vi "Hydra.vi"() -> ()   [LabVIEW 2019]
uses:
  Global Variables/Global_Variables.vi
panel:
  in  "Press Transducer Cal":u16(ring) items=["Low Pressure", "High Pressure"]
  in  "Cal Add":bool
  out "Error Code":i32
  out "Error Description":string
  out "Data":string[][](table)
  in  "Check":bool
  in  "Start Test":bool
  in  "Stop Test":bool
  in  "Quit":bool
  out "Channel_Config":string[][](table)
  in  "Add Button":bool
  in  "Cal":bool
  in  "Range":u16(ring)
  in  "Type":u16(ring)
  in  "Name":string
  in  "Channel":u16(ring)
  out "Status":string
  in  "Test Name":string
  in  "COM Port - Hydra":refnum<visa-resource-name>
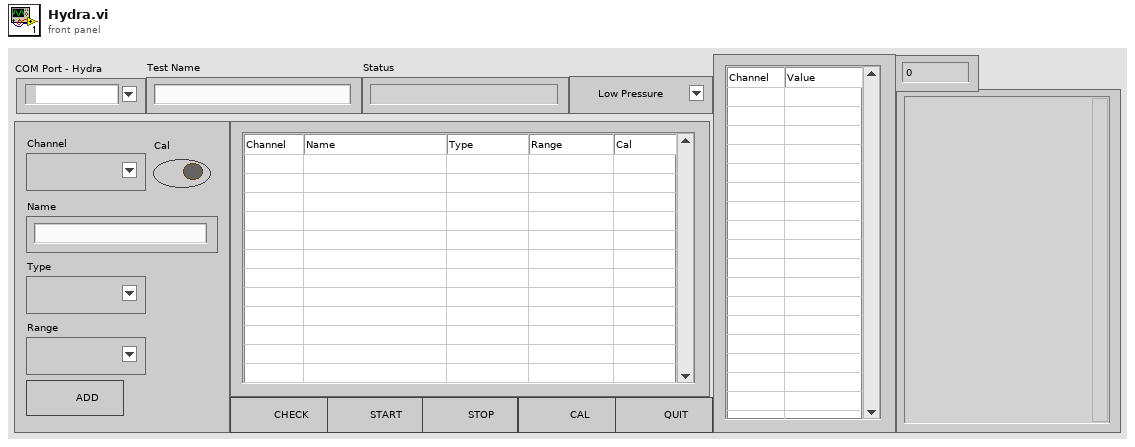
[diagram p1: front panel]
types:
  T1 = enum16{"Initialize", "Wait for Config", "Calibration", "Test", "Close"}
  T2 = enum8{"Enabled", "Disabled", "Disabled and Grayed Out"}
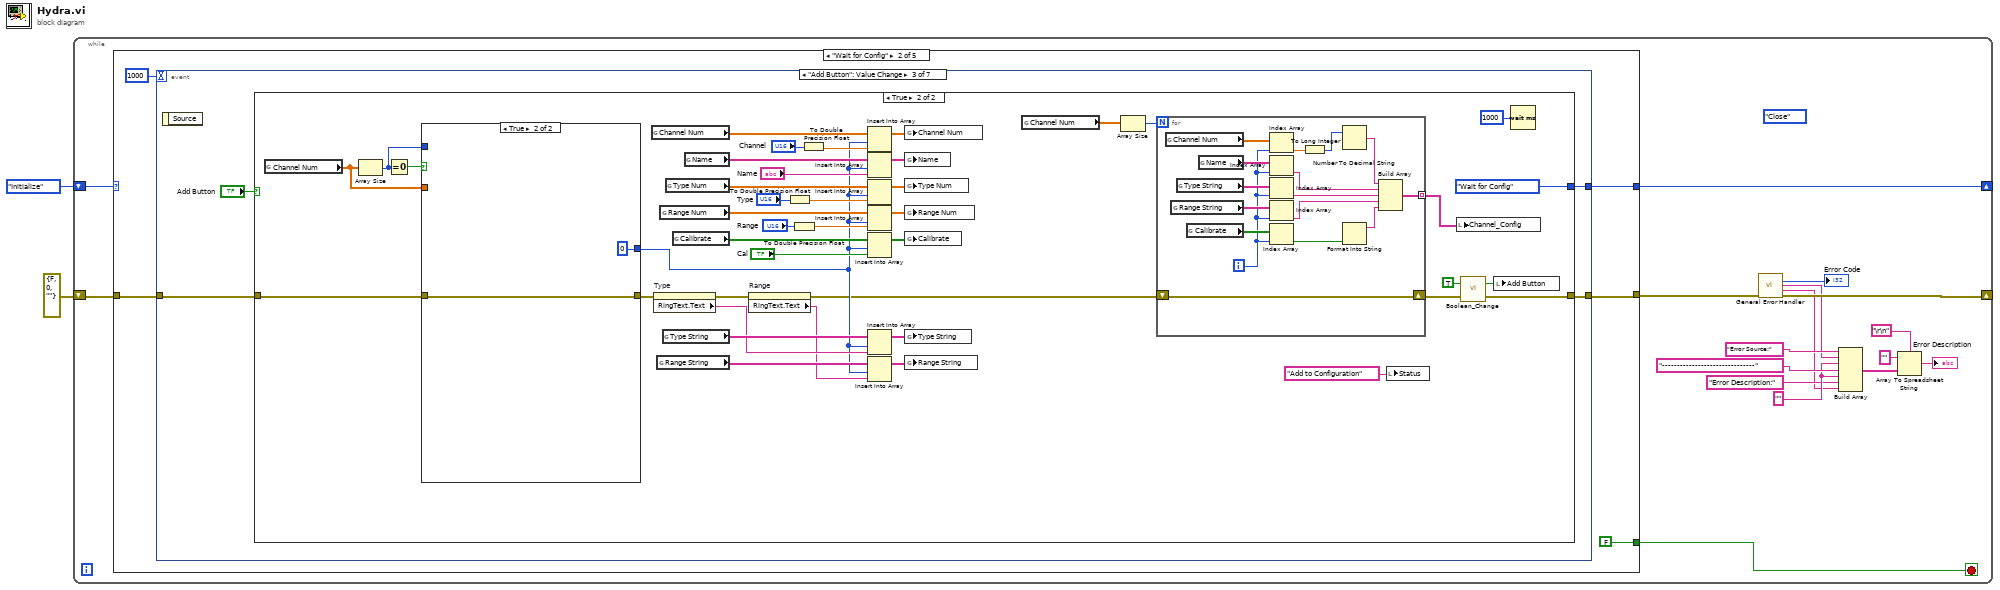
[diagram p0: block diagram]
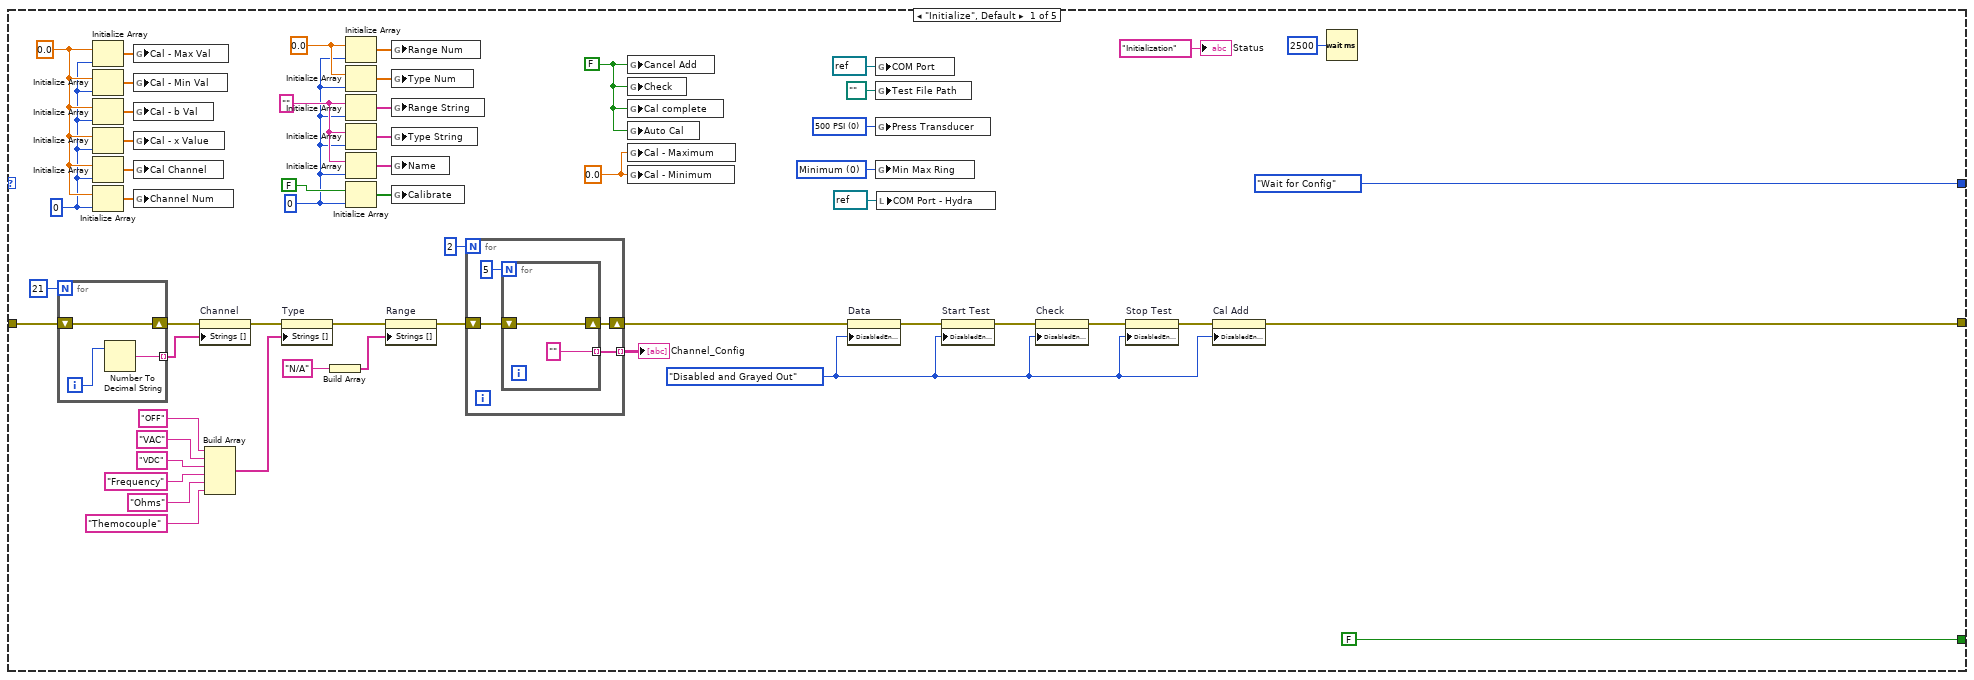
[diagram p2: hidden frame]
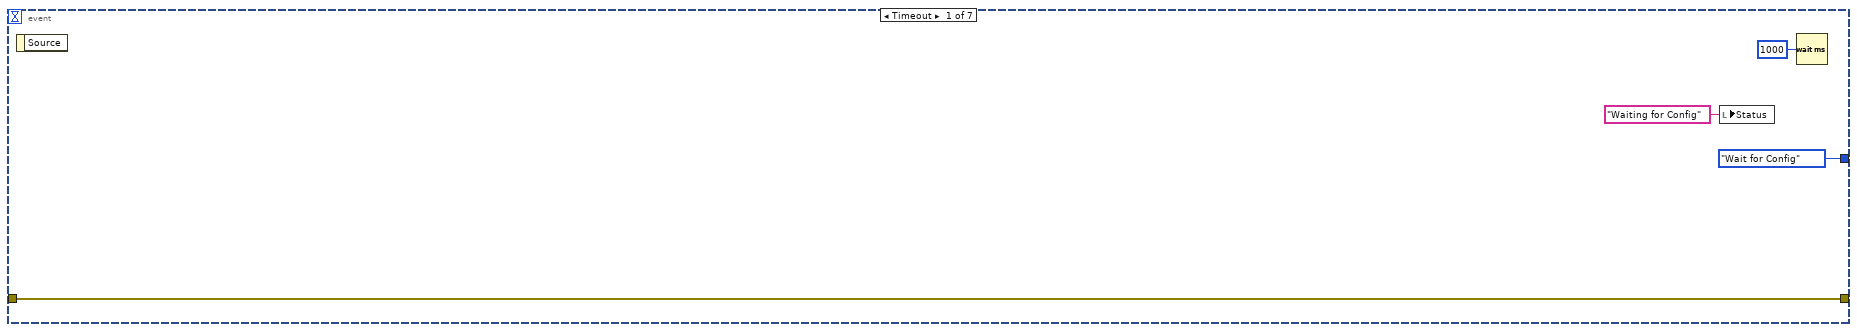
[diagram p3: hidden frame]
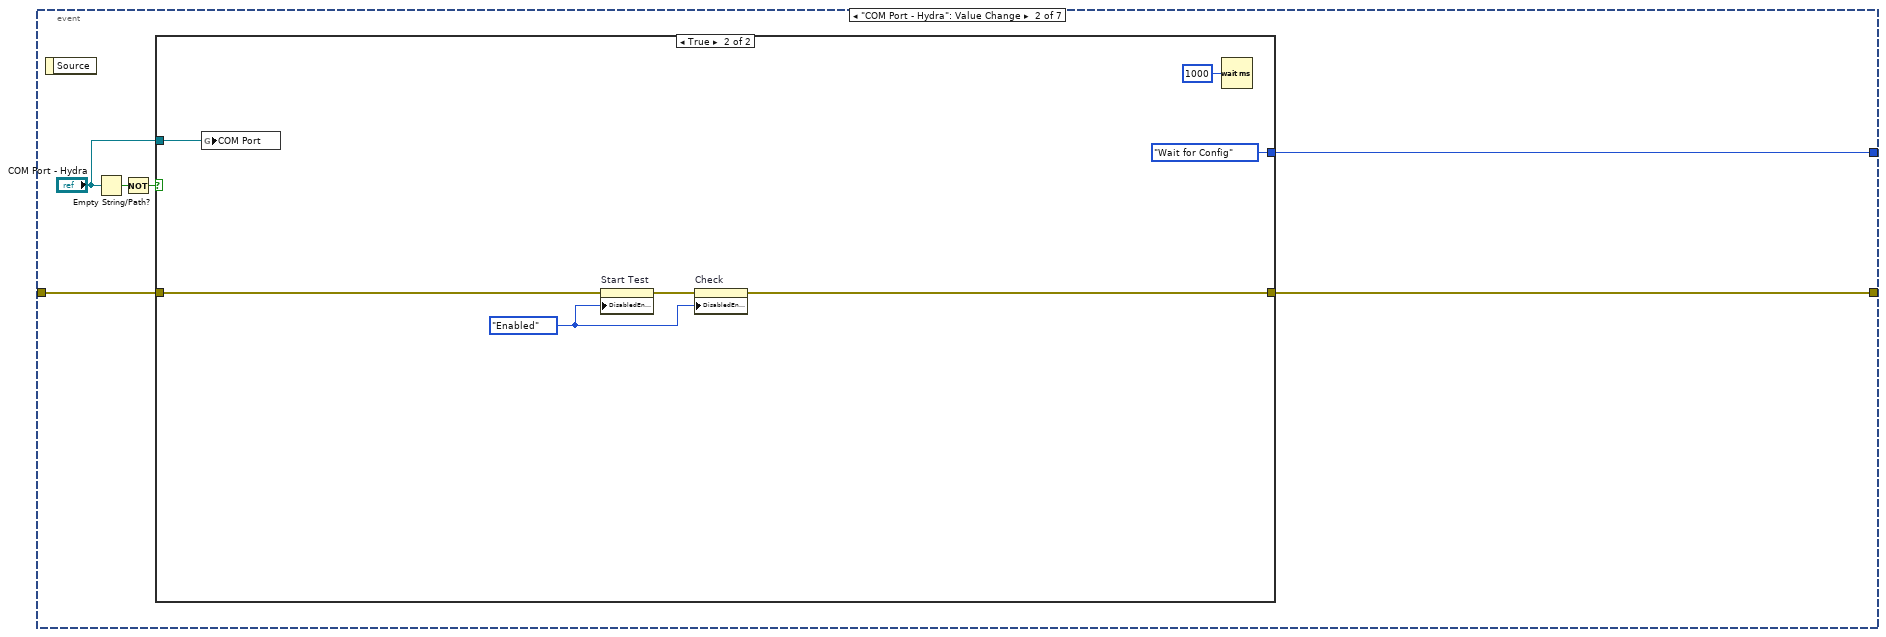
[diagram p4: hidden frame]
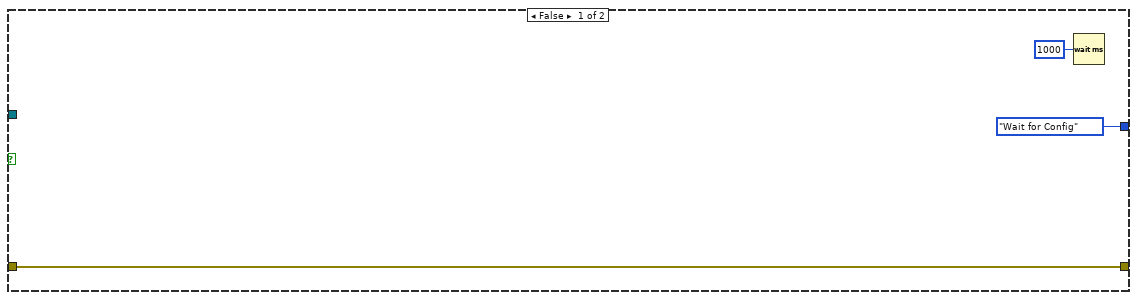
[diagram p5: hidden frame]
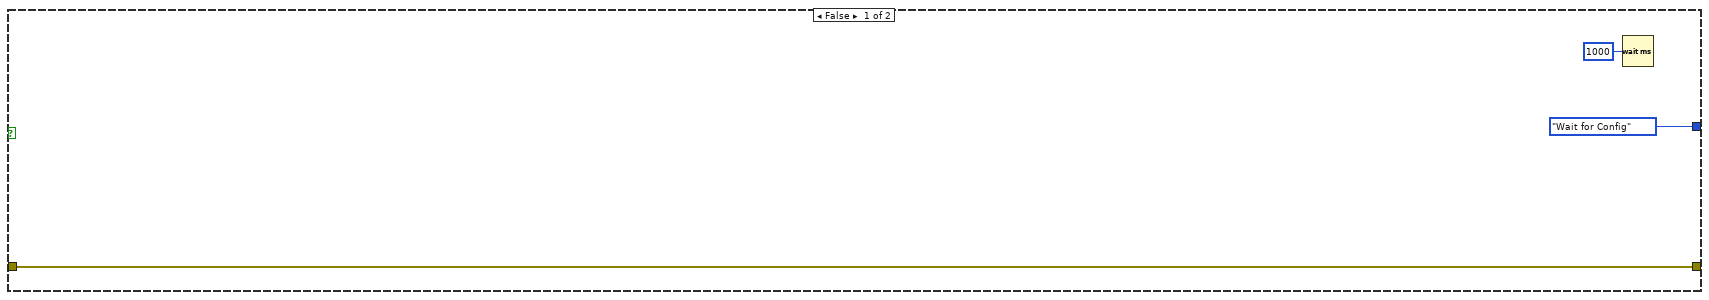
[diagram p6: hidden frame]
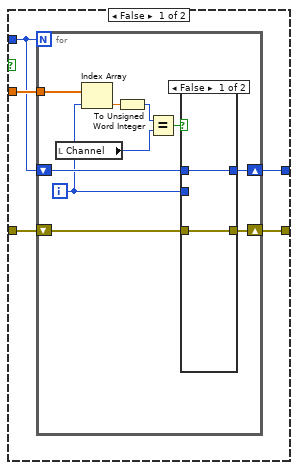
[diagram p7: hidden frame]
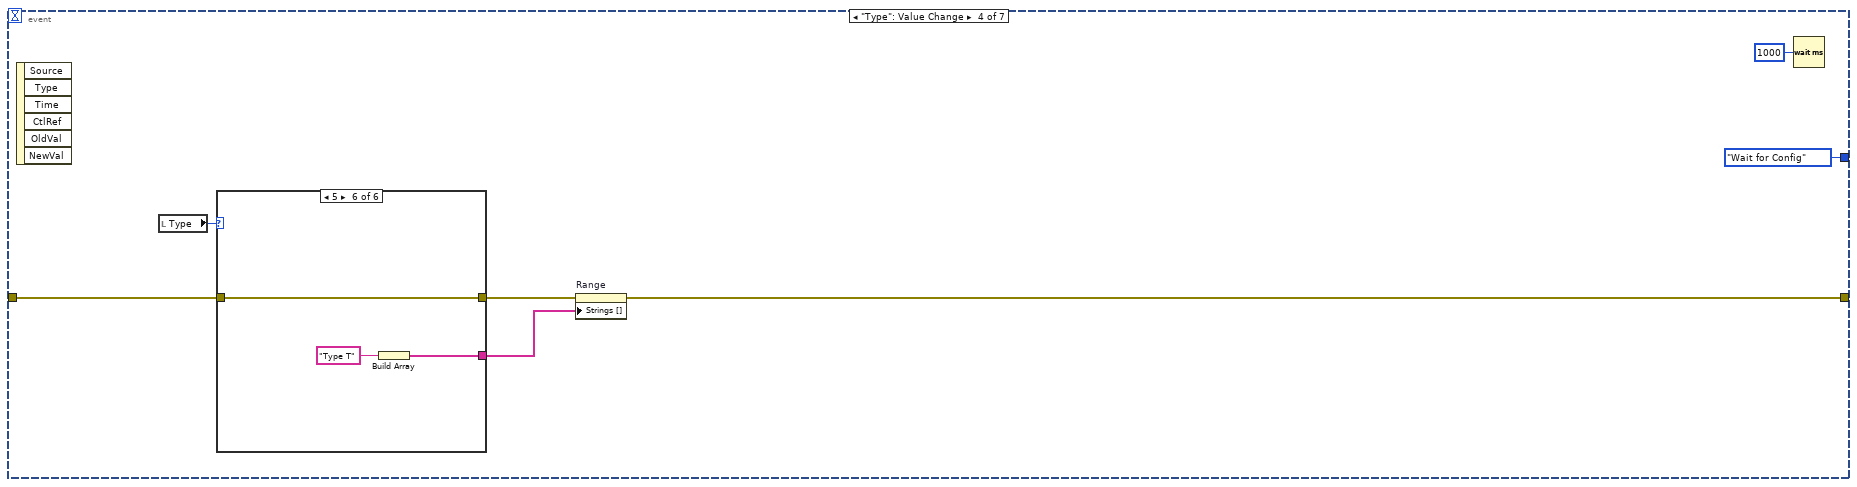
[diagram p9: hidden frame]
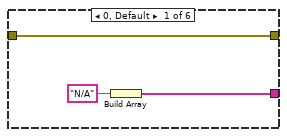
[diagram p10: hidden frame]
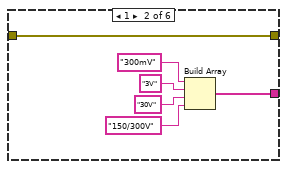
[diagram p11: hidden frame]
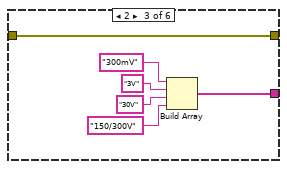
[diagram p12: hidden frame]
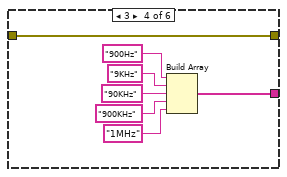
[diagram p13: hidden frame]
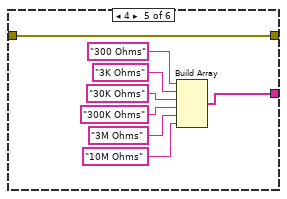
[diagram p14: hidden frame]
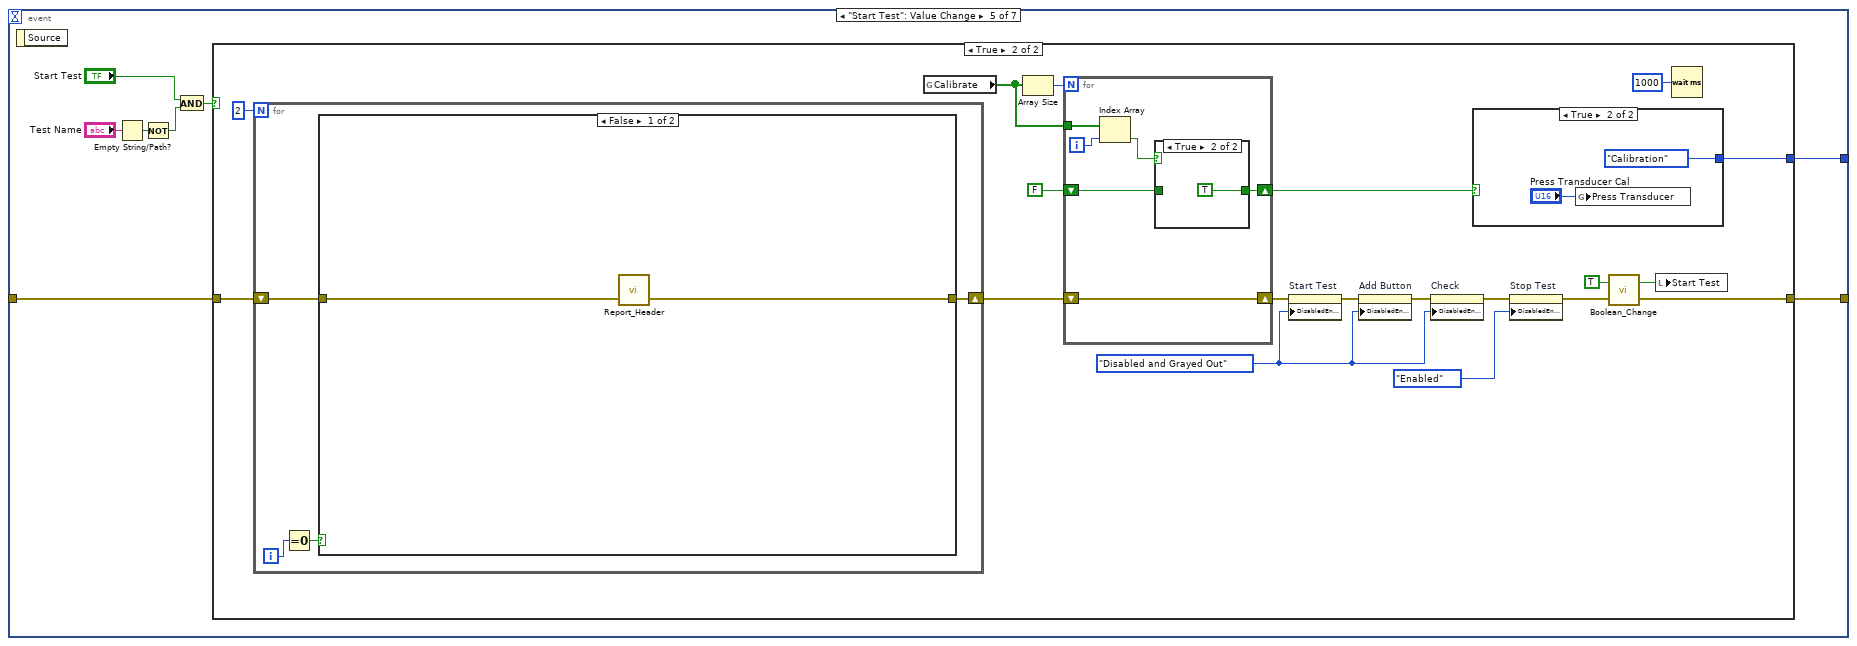
[diagram p15: hidden frame]
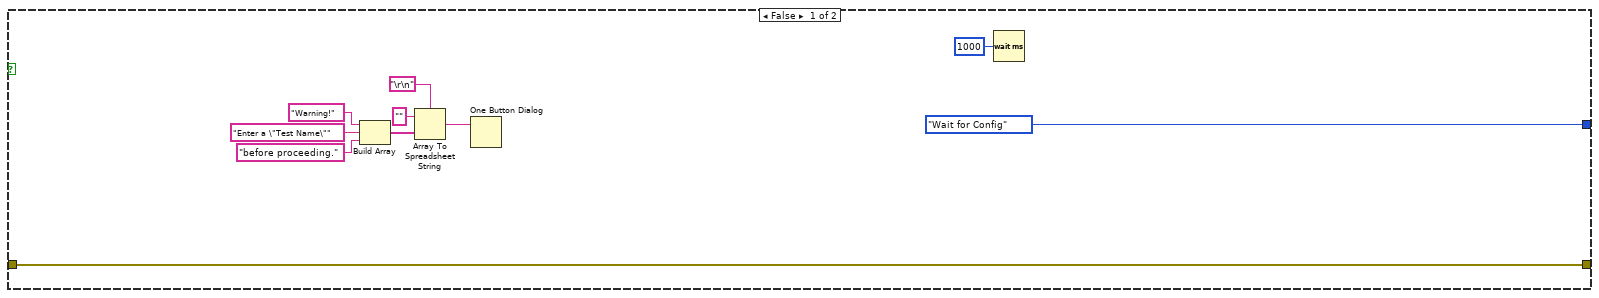
[diagram p16: hidden frame]
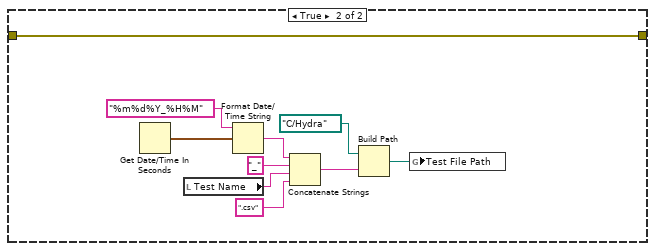
[diagram p17: hidden frame]
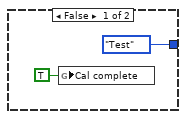
[diagram p18: hidden frame]
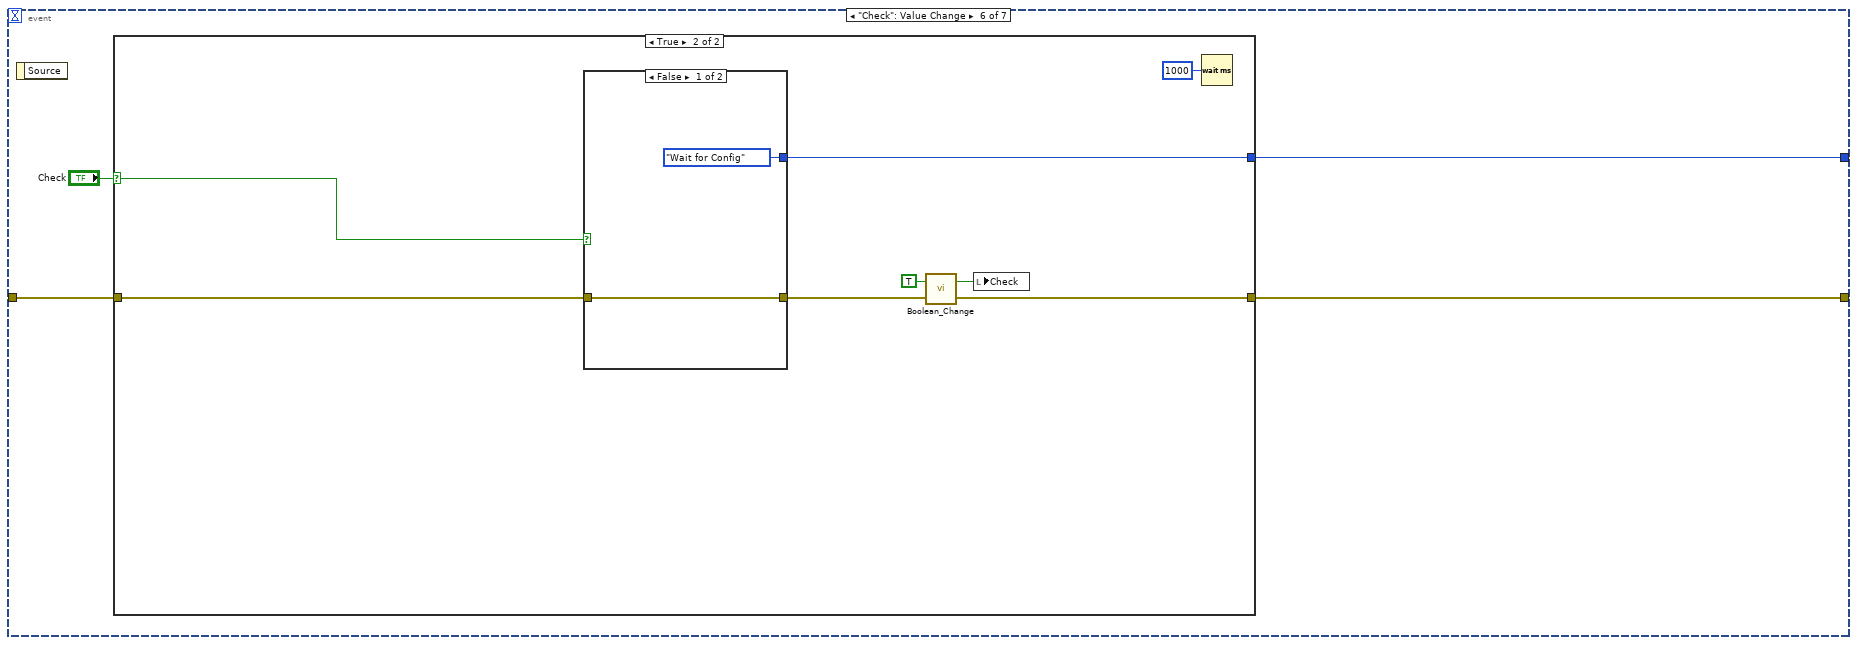
[diagram p20: hidden frame]
diagram:
  n1 = while {
    shift-right: [w15] -> _
    shift-left: errorcluster {"status"=FALSE, "code"=0, "source"=""} ("error constant") -> [w18]
    shift-right: [w3] -> _
    shift-left: T1."Initialize" -> [w19]
    stop <- w17 stop-if-true
    (unwired) T1."Close"
    w10 = ""
    n2 = case shown="\"Wait for Config\"" w19 {
      tunnel: w18 -> [w70 w86 w333 w594 w629]
      tunnel: [w45 w83 w331 w593 w629] -> w16
      tunnel: [FALSE FALSE FALSE FALSE TRUE] -> w17
      tunnel: [T1."Wait for Config" w84 w330 w592 T1."Close"] -> w3
      frame "Initialize", Default {
        w21 = u16 0 items=["Minimum", "Maximum"] ("Min Max Ring")
        w22 = u16 0 items=["500 PSI", "1000 PSI"] ("Press Transducer")
        w25 = FALSE ("Cancel Add")
        w26 = 0.0 ("Cal - Minimum")
        w34 = ""
        w36 = 0.0 ("element")
        w33 = 0 ("dimension size")
        w43 = 0 ("dimension size")
        w44 = 0.0 ("element")
        w46 = T2."Disabled and Grayed Out" ("Disabled")
        n3 = for {
          N: 21 -> [_]
          shift-right: [w82] -> w69
          shift-left: w70 -> [w82]
          tunnel: [w80] -> w68 mode=indexing
          i -> [w81]
          n4 = Number To Decimal String(number=w81) -> (decimal integer string=w80:string)  [unwired: 1 in]
        }
        n5 = Initialize Array(w44, w43) -> (w42:dbl[])
        n6 = Initialize Array(w44, w43) -> (w41:dbl[])
        n7 = Initialize Array(w44, w43) -> (w40:dbl[])
        n8 = Initialize Array(w44, w43) -> (w39:dbl[])
        n9 = Initialize Array(w44, w43) -> (w38:dbl[])
        n10 = Initialize Array(w44, w43) -> (w37:dbl[])
        n11 = global write "Global_Variables.vi" "Cal - Max Val"(w42) -> ()
        n12 = global write "Global_Variables.vi" "Cal - Min Val"(w41) -> ()
        n13 = global write "Global_Variables.vi" "Cal - b Val"(w40) -> ()
        n14 = global write "Global_Variables.vi" "Cal - x Value"(w39) -> ()
        n15 = global write "Global_Variables.vi" "Cal Channel"(w38) -> ()
        n16 = global write "Global_Variables.vi" "Channel Num"(w37) -> ()
        n17 = property on="Channel" class="Ring (strict)"(error in=w69, "Strings []"=w68) -> (error out=w61:errorcluster)  [unwired: 1 in, 1 out]
        n18 = Build Array("OFF", "VAC", "VDC", "Frequency", "Ohms", "Themocouple") -> (w60:string[])
        n19 = property on="Type" class="Ring (strict)"(error in=w61, "Strings []"=w60) -> (error out=w59:errorcluster)  [unwired: 1 in, 1 out]
        n20 = Build Array("N/A") -> (w57:string[])
        n21 = Initialize Array(w36, w33) -> (w32:dbl[])
        n22 = Initialize Array(w36, w33) -> (w31:dbl[])
        n23 = Initialize Array(w34, w33) -> (w30:string[])
        n24 = Initialize Array(w34, w33) -> (w29:string[])
        n25 = Initialize Array(w34, w33) -> (w28:string[])
        n26 = Initialize Array(FALSE, w33) -> (w27:bool[])
        n27 = property on="Range" class="Ring (strict)"(error in=w59, "Strings []"=w57) -> (error out=w56:errorcluster)  [unwired: 1 in, 1 out]
        n28 = global write "Global_Variables.vi" "Range Num"(w32) -> ()
        n29 = global write "Global_Variables.vi" "Type Num"(w31) -> ()
        n30 = global write "Global_Variables.vi" "Range String"(w30) -> ()
        n31 = global write "Global_Variables.vi" "Type String"(w29) -> ()
        n32 = global write "Global_Variables.vi" "Name"(w28) -> ()
        n33 = global write "Global_Variables.vi" "Calibrate"(w27) -> ()
        n34 = for {
          N: 2 -> [_]
          shift-right: [w75] -> w53
          shift-left: w56 -> [w76]
          tunnel: [w74] -> w54 mode=indexing
          n35 = for {
            N: 5 -> [_]
            shift-right: [w79] -> w75
            shift-left: w76 -> [w79]
            tunnel: [""] -> w74 mode=indexing
          }
        }
        "Channel_Config" <- w54
        n36 = global write "Global_Variables.vi" "Cancel Add"(w25) -> ()
        n37 = global write "Global_Variables.vi" "Check"(w25) -> ()
        n38 = global write "Global_Variables.vi" "Cal complete"(w25) -> ()
        n39 = global write "Global_Variables.vi" "Auto Cal"(w25) -> ()
        n40 = global write "Global_Variables.vi" "Cal - Maximum"(w26) -> ()
        n41 = global write "Global_Variables.vi" "Cal - Minimum"(w26) -> ()
        n42 = property on="Data" class="Tbl (strict)"(error in=w53, "DisabledEnum"=w46) -> (error out=w52:errorcluster)  [unwired: 1 in, 1 out]
        n43 = global write "Global_Variables.vi" "COM Port"(refnum<visa-resource-name> refnum ("COM Port")) -> ()
        n44 = global write "Global_Variables.vi" "Test File Path"(path "" ("Test File Path")) -> ()
        n45 = global write "Global_Variables.vi" "Press Transducer"(w22) -> ()
        n46 = global write "Global_Variables.vi" "Min Max Ring"(w21) -> ()
        n47 = local write "COM Port - Hydra"(refnum<visa-resource-name> refnum ("COM Port - Hydra")) -> ()
        n48 = property on="Start Test" class="Bool (strict)"(error in=w52, "DisabledEnum"=w46) -> (error out=w51:errorcluster)  [unwired: 1 in, 1 out]
        n49 = property on="Check" class="Bool (strict)"(error in=w51, "DisabledEnum"=w46) -> (error out=w50:errorcluster)  [unwired: 1 in, 1 out]
        n50 = property on="Stop Test" class="Bool (strict)"(error in=w50, "DisabledEnum"=w46) -> (error out=w47:errorcluster)  [unwired: 1 in, 1 out]
        n51 = property on="Cal Add" class="Bool (strict)"(error in=w47, "DisabledEnum"=w46) -> (error out=w45:errorcluster)  [unwired: 1 in, 1 out]
        n52 = Wait (ms)(milliseconds to wait=u32 2500) -> ()  [unwired: 1 out]
        "Status" <- "Initialization" ("Status")
      }
      frame "Wait for Config" {
        n53 = event shown="[2] \"Add Button\": Value Change" {
          selector: _ -> [_ _ _ _ _ _ _]
          dyn-events: _ -> [_ _ _ _ _ _ _]
          timeout: 1000 -> [_ _ _ _ _ _ _]
          tunnel: w86 -> [w91 w96 w110 w199 w237 w300 w321]
          tunnel: [T1."Wait for Config" w97 w108 T1."Wait for Config" w236 w301 w320] -> w84
          tunnel: [w91 w95 w109 w195 w234 w299 w319] -> w83
          event Timeout {
            n54 = event-data() -> ()  [unwired: 1 in, 1 out]
            n55 = local write "Status"("Waiting for Config" ("Status")) -> ()
            n56 = Wait (ms)(milliseconds to wait=u32 1000) -> ()  [unwired: 1 out]
          }
          event "COM Port - Hydra": Value Change {
            n57 = event-data() -> ()  [unwired: 1 in, 1 out]
            n58 = Empty String/Path?(string/path="COM Port - Hydra") -> (empty?=w93:bool)
            n59 = Not(x=w93) -> (.not. x?=w92:bool)
            n60 = case shown="True" w92 {
              tunnel: [T1."Wait for Config" T1."Wait for Config"] -> w97
              tunnel: w96 -> [w99 w107]
              tunnel: [w99 w105] -> w95
              tunnel: "COM Port - Hydra" -> [_ w101]
              frame False {
                n61 = Wait (ms)(milliseconds to wait=u32 1000) -> ()  [unwired: 1 out]
              }
              frame True {
                w103 = T2."Enabled" ("Disabled")
                n62 = global write "Global_Variables.vi" "COM Port"(w101) -> ()
                n63 = property on="Start Test" class="Bool (strict)"(error in=w107, "DisabledEnum"=w103) -> (error out=w106:errorcluster)  [unwired: 1 in, 1 out]
                n64 = property on="Check" class="Bool (strict)"(error in=w106, "DisabledEnum"=w103) -> (error out=w105:errorcluster)  [unwired: 1 in, 1 out]
                n65 = Wait (ms)(milliseconds to wait=u32 1000) -> ()  [unwired: 1 out]
              }
            }
          }
          event "Add Button": Value Change {
            n66 = event-data() -> ()  [unwired: 1 in, 1 out]
            n67 = case shown="True" "Add Button" {
              tunnel: w110 -> [w114 w154]
              tunnel: [w114 w117] -> w109
              tunnel: [T1."Wait for Config" T1."Wait for Config"] -> w108
              frame False {
                n68 = Wait (ms)(milliseconds to wait=u32 1000) -> ()  [unwired: 1 out]
              }
              frame True {
                n69 = global read "Global_Variables.vi" "Channel Num"() -> (w155:dbl[])
                n70 = Array Size(array=w155) -> (size(s)=w153:i32)
                n71 = Equal To 0?(x=w153) -> (x = 0?=w156:bool)
                n72 = case shown="True" w156 {
                  tunnel: w155 -> [w177 _]
                  tunnel: w154 -> [w176 w193]
                  tunnel: [w175 w193] -> w144
                  tunnel: w153 -> [w173 _]
                  tunnel: [w174 0] -> w131
                  frame False {
                    n73 = for {
                      N: w173 -> [_]
                      tunnel: w177 -> [w187]
                      shift-right: [w181] -> w175
                      shift-left: w176 -> [w182]
                      shift-right: [w179] -> w174
                      shift-left: w173 -> [w180]
                      i -> [w178]
                      n74 = local read "Channel"() -> (w184:u16)
                      n75 = Index Array(array=w187, index=w178) -> (element=w186:dbl)
                      n76 = To Unsigned Word Integer(number=w186) -> (unsigned 16bit integer=w185:u16)
                      n77 = Equal?(x=w185, y=w184) -> (x = y?=w183:bool)
                      n78 = case shown="False" w183 {
                        tunnel: w182 -> [w188 w191]
                        tunnel: [w188 w191] -> w181
                        tunnel: w180 -> [w189 _]
                        tunnel: [w189 w190] -> w179
                        tunnel: w178 -> [_ w190]
                        frame False {
                        }
                        frame True {
                        }
                      }
                    }
                  }
                  frame True {
                  }
                }
                n79 = global read "Global_Variables.vi" "Channel Num"() -> (w150:dbl[])
                n80 = property on="Type" class="Ring (strict)"(error in=w144) -> (error out=w143:errorcluster, "RingText.Text"=w133:string)  [unwired: 1 in, 1 out]
                n81 = global read "Global_Variables.vi" "Range String"() -> (w146:string[])
                n82 = global read "Global_Variables.vi" "Range Num"() -> (w148:dbl[])
                n83 = global read "Global_Variables.vi" "Type String"() -> (w145:string[])
                n84 = global read "Global_Variables.vi" "Type Num"() -> (w142:dbl[])
                n85 = global read "Global_Variables.vi" "Calibrate"() -> (w147:bool[])
                n86 = global read "Global_Variables.vi" "Name"() -> (w149:string[])
                n87 = property on="Range" class="Ring (strict)"(error in=w143) -> (error out=w121:errorcluster, "RingText.Text"=w132:string)  [unwired: 1 in, 1 out]
                n88 = To Double Precision Float(number="Type") -> (double precision float=w137:dbl)
                n89 = To Double Precision Float(number="Range") -> (double precision float=w135:dbl)
                n90 = To Double Precision Float(number="Channel") -> (double precision float=w140:dbl)
                n91 = Insert Into Array(array=w150, index=w131, new element=w140) -> (w127:dbl[])
                n92 = Insert Into Array(array=w149, index=w131, new element="Name") -> (w126:string[])
                n93 = Insert Into Array(array=w142, index=w131, new element=w137) -> (w125:dbl[])
                n94 = Insert Into Array(array=w148, index=w131, new element=w135) -> (w124:dbl[])
                n95 = Insert Into Array(array=w147, index=w131, new element="Cal") -> (w128:bool[])
                n96 = Insert Into Array(array=w145, index=w131, new element=w133) -> (w129:string[])
                n97 = Insert Into Array(array=w146, index=w131, new element=w132) -> (w130:string[])
                n98 = global write "Global_Variables.vi" "Channel Num"(w127) -> ()
                n99 = global write "Global_Variables.vi" "Name"(w126) -> ()
                n100 = global write "Global_Variables.vi" "Type Num"(w125) -> ()
                n101 = global write "Global_Variables.vi" "Range Num"(w124) -> ()
                n102 = global write "Global_Variables.vi" "Calibrate"(w128) -> ()
                n103 = global write "Global_Variables.vi" "Type String"(w129) -> ()
                n104 = global write "Global_Variables.vi" "Range String"(w130) -> ()
                n105 = global read "Global_Variables.vi" "Channel Num"() -> (w123:dbl[])
                n106 = Array Size(array=w123) -> (size(s)=w122:i32)
                n107 = for {
                  N: w122 -> [_]
                  shift-right: [w167] -> w118
                  shift-left: w121 -> [w167]
                  tunnel: [w160] -> w120 mode=indexing
                  i -> [w157]
                  n108 = global read "Global_Variables.vi" "Channel Num"() -> (w168:dbl[])
                  n109 = global read "Global_Variables.vi" "Range String"() -> (w171:string[])
                  n110 = global read "Global_Variables.vi" "Type String"() -> (w170:string[])
                  n111 = global read "Global_Variables.vi" "Calibrate"() -> (w172:bool[])
                  n112 = global read "Global_Variables.vi" "Name"() -> (w169:string[])
                  n113 = Index Array(array=w168, index=w157) -> (element=w166:dbl)
                  n114 = Index Array(array=w169, index=w157) -> (element=w158:string)
                  n115 = Index Array(array=w170, index=w157) -> (element=w161:string)
                  n116 = Index Array(array=w171, index=w157) -> (element=w159:string)
                  n117 = Index Array(array=w172, index=w157) -> (element=w164:bool)
                  n118 = To Long Integer(number=w166) -> (32bit integer=w165:i32)
                  n119 = Number To Decimal String(number=w165) -> (decimal integer string=w163:string)  [unwired: 1 in]
                  n120 = Format Into String(w164) -> (resulting string=w162:string)  [unwired: 3 in, 1 out]
                  n121 = Build Array(w163, w158, w161, w159, w162) -> (w160:string[])
                }
                n122 = local write "Status"("Add to Configuration" ("Status")) -> ()
                n123 = local write "Channel_Config"(w120) -> ()
                n124 = call "Boolean_Change.vi"("Error In"=w118, "Input"=TRUE) -> ("Error Out"=w117:errorcluster, "Output"=w115:bool)
                n125 = local write "Add Button"(w115) -> ()
                n126 = Wait (ms)(milliseconds to wait=u32 1000) -> ()  [unwired: 1 out]
              }
            }
          }
          event "Type": Value Change {
            n127 = event-data() -> ()  [unwired: 1 in, 6 out]
            n128 = local read "Type"() -> (w200:u16)
            n129 = case shown="5" w200 {
              tunnel: w199 -> [w202 w209 w215 w222 w230 w233]
              tunnel: [w202 w209 w215 w222 w230 w233] -> w196
              tunnel: [w201 w204 w210 w216 w223 w231] -> w194
              frame 0, Default {
                n130 = Build Array("N/A") -> (w201:string[])
              }
              frame 1 {
                n131 = Build Array("300mV", "3V", "30V", "150/300V") -> (w204:string[])
              }
              frame 2 {
                n132 = Build Array("300mV", "3V", "30V", "150/300V") -> (w210:string[])
              }
              frame 3 {
                n133 = Build Array("900Hz", "9KHz", "90KHz", "900KHz", "1MHz") -> (w216:string[])
              }
              frame 4 {
                n134 = Build Array("300 Ohms", "3K Ohms", "30K Ohms", "300K Ohms", "3M Ohms", "10M Ohms") -> (w223:string[])
              }
              frame 5 {
                n135 = Build Array("Type T") -> (w231:string[])
              }
            }
            n136 = property on="Range" class="Ring (strict)"(error in=w196, "Strings []"=w194) -> (error out=w195:errorcluster)  [unwired: 1 in, 1 out]
            n137 = Wait (ms)(milliseconds to wait=u32 1000) -> ()  [unwired: 1 out]
          }
          event "Start Test": Value Change {
            n138 = event-data() -> ()  [unwired: 1 in, 1 out]
            n139 = Empty String/Path?(string/path="Test Name") -> (empty?=w240:bool)
            n140 = Not(x=w240) -> (.not. x?=w235:bool)
            n141 = And(x="Start Test", y=w235) -> (x .and. y?=w238:bool)
            n142 = case shown="True" w238 {
              tunnel: w237 -> [w250 w253]
              tunnel: [T1."Wait for Config" w255] -> w236
              tunnel: [w250 w266] -> w234
              frame False {
                n143 = Build Array("Warning!" ("message"), "Enter a \"Test Name\"", "before proceeding.") -> (w245:string[])
                n144 = Array To Spreadsheet String(delimiter (Tab)="\r\n", array=w245, 3:"" ("format string")) -> (spreadsheet string=w242:string)
                n145 = One Button Dialog(message=w242) -> ()  [unwired: 1 in, 1 out]
                n146 = Wait (ms)(milliseconds to wait=u32 1000) -> ()  [unwired: 1 out]
              }
              frame True {
                w262 = T2."Disabled and Grayed Out" ("Disabled")
                n147 = for {
                  N: 2 -> [_]
                  shift-right: [w271] -> w252
                  shift-left: w253 -> [w272]
                  i -> [w274]
                  n148 = Equal To 0?(x=w274) -> (x = 0?=w273:bool)
                  n149 = case shown="False" w273 {
                    tunnel: w272 -> [w276 w278]
                    tunnel: [w275 w278] -> w271
                    frame False {
                      n150 = call "Report_Header.vi"("Error In"=w276) -> ("Error Out"=w275:errorcluster)  [unwired: 2 in]
                    }
                    frame True {
                      n151 = Get Date/Time In Seconds() -> (seconds since 1Jan1904=w283:timestamp)
                      n152 = local read "Test Name"() -> (w285:string)
                      n153 = Format Date/Time String(time format string (%c)="%m%d%Y_%H%M", seconds (now)=w283) -> (date/time string=w284:string)  [unwired: 1 in]
                      n154 = Concatenate Strings(w284, "_", w285, ".csv") -> (w286:string)
                      n155 = Build Path(base path=path "C:/Hydra", name or relative path=w286) -> (appended path=w277:path)
                      n156 = global write "Global_Variables.vi" "Test File Path"(w277) -> ()
                    }
                  }
                }
                n157 = global read "Global_Variables.vi" "Calibrate"() -> (w258:bool[])
                n158 = Array Size(array=w258) -> (size(s)=w259:i32)
                n159 = for {
                  N: w259 -> [_]
                  shift-right: [w296] -> w260
                  shift-left: w252 -> [w296]
                  tunnel: w258 -> [w295]
                  shift-right: [w291] -> w256
                  shift-left: FALSE -> [w292]
                  i -> [w294]
                  n160 = Index Array(array=w295, index=w294) -> (element=w293:bool)
                  n161 = case shown="True" w293 {
                    tunnel: w292 -> [w297 _]
                    tunnel: [w297 TRUE] -> w291
                    frame False {
                    }
                    frame True {
                    }
                  }
                }
                n162 = property on="Start Test" class="Bool (strict)"(error in=w260, "DisabledEnum"=w262) -> (error out=w269:errorcluster)  [unwired: 1 in, 1 out]
                n163 = property on="Add Button" class="Bool (strict)"(error in=w269, "DisabledEnum"=w262) -> (error out=w268:errorcluster)  [unwired: 1 in, 1 out]
                n164 = property on="Check" class="Bool (strict)"(error in=w268, "DisabledEnum"=w262) -> (error out=w264:errorcluster)  [unwired: 1 in, 1 out]
                n165 = case shown="True" w256 {
                  tunnel: [T1."Test" T1."Calibration"] -> w255
                  frame False {
                    n166 = global write "Global_Variables.vi" "Cal complete"(TRUE ("Cal complete")) -> ()
                  }
                  frame True {
                    n167 = global write "Global_Variables.vi" "Press Transducer"("Press Transducer Cal") -> ()
                  }
                }
                n168 = property on="Stop Test" class="Bool (strict)"(error in=w264, "DisabledEnum"=T2."Enabled" ("Disabled")) -> (error out=w263:errorcluster)  [unwired: 1 in, 1 out]
                n169 = call "Boolean_Change.vi"("Error In"=w263, "Input"=TRUE) -> ("Error Out"=w266:errorcluster, "Output"=w265:bool)
                n170 = local write "Start Test"(w265) -> ()
                n171 = Wait (ms)(milliseconds to wait=u32 1000) -> ()  [unwired: 1 out]
              }
            }
          }
          event "Check": Value Change {
            n172 = event-data() -> ()  [unwired: 1 in, 1 out]
            n173 = case shown="True" "Check" {
              selector: "Check" -> [_ w312]
              tunnel: [T1."Wait for Config" w310] -> w301
              tunnel: w300 -> [w303 w311]
              tunnel: [w303 w307] -> w299
              frame False {
                n174 = Wait (ms)(milliseconds to wait=u32 1000) -> ()  [unwired: 1 out]
              }
              frame True {
                n175 = case shown="False" w312 {
                  tunnel: w311 -> [w315 w318]
                  tunnel: [w315 w318] -> w309
                  tunnel: [T1."Wait for Config" T1."Test"] -> w310
                  frame False {
                  }
                  frame True {
                    n176 = global write "Global_Variables.vi" "Check"(TRUE ("Check")) -> ()
                  }
                }
                n177 = call "Boolean_Change.vi"("Error In"=w309, "Input"=TRUE) -> ("Error Out"=w307:errorcluster, "Output"=w306:bool)
                n178 = local write "Check"(w306) -> ()
                n179 = Wait (ms)(milliseconds to wait=u32 1000) -> ()  [unwired: 1 out]
              }
            }
          }
          event "Quit": Value Change {
            n180 = event-data() -> ()  [unwired: 1 in, 1 out]
            n181 = case shown="False" "Quit" {
              tunnel: w321 -> [w324 w326]
              tunnel: [T1."Wait for Config" T1."Close"] -> w320
              tunnel: [w324 w326] -> w319
              frame False {
                n182 = Wait (ms)(milliseconds to wait=u32 1000) -> ()  [unwired: 1 out]
              }
              frame True {
              }
            }
          }
        }
      }
      frame "Calibration" {
        n183 = feedback #1(enum16{"Minimum", "Maximum", "Calculations"}."Minimum") -> (w334:enum16{"Minimum", "Maximum", "Calculations"})
        n184 = case shown="\"Minimum\", Default" w334 {
          selector: w334 -> [w337 w479 _]
          tunnel: w333 -> [w339 w478 w588]
          tunnel: [w340 w475 enum16{"Minimum", "Maximum", "Calculations"}."Minimum"] -> w332
          tunnel: [w338 w477 w587] -> w331
          tunnel: [w336 w476 T1."Test"] -> w330
          frame "Minimum", Default {
            n185 = event shown="[1] \"Cal Add\": Value Change" {
              selector: _ -> [_ _]
              dyn-events: _ -> [_ _]
              timeout: 1000 -> [_ _]
              tunnel: [w346 w399] -> w340
              tunnel: w339 -> [w354 w401]
              tunnel: [w348 w400] -> w338
              tunnel: w337 -> [w346 w397]
              tunnel: [T1."Calibration" w398] -> w336
              event Timeout {
                n186 = event-data() -> ()  [unwired: 1 in, 1 out]
                n187 = feedback #2(0) -> (w343:i32)
                n188 = case shown="0, Default" w343 {
                  selector: w343 -> [w356 w378]
                  tunnel: w354 -> [w358 w379]
                  tunnel: [w357 w379] -> w352
                  tunnel: [w355 w378] -> w342
                  frame 0, Default {
                    n189 = global read "Global_Variables.vi" "Calibrate"() -> (w360:bool[])
                    n190 = Array Size(array=w360) -> (size(s)=w359:i32)
                    n191 = for {
                      N: w359 -> [_]
                      shift-right: [w362] -> w357
                      shift-left: w358 -> [w363]
                      i -> [w361]
                      n192 = global read "Global_Variables.vi" "Calibrate"() -> (w365:bool[])
                      n193 = Index Array(array=w365, index=w361) -> (element=w364:bool)
                      n194 = case shown="True" w364 {
                        tunnel: w363 -> [w366 w376]
                        tunnel: [w366 w376] -> w362
                        tunnel: w361 -> [_ w374]
                        frame False {
                        }
                        frame True {
                          n195 = global read "Global_Variables.vi" "Cal Channel"() -> (w372:dbl[])
                          n196 = global read "Global_Variables.vi" "Channel Num"() -> (w375:dbl[])
                          n197 = Array Size(array=w372) -> (size(s)=w373:i32)
                          n198 = Index Array(array=w375, index=w374) -> (element=w368:dbl)
                          n199 = Insert Into Array(array=w372, index=w373, new element=w368) -> (w371:dbl[])
                          n200 = To Long Integer(number=w368) -> (32bit integer=w369:i32)
                          n201 = Equal?(x=w369, y=0) -> (x = y?=w370:bool)
                          n202 = global write "Global_Variables.vi" "Cal Channel"(w371) -> ()
                          n203 = case shown="True" w370 {
                            frame False {
                            }
                            frame True {
                              n204 = global write "Global_Variables.vi" "Auto Cal"(TRUE ("Auto Cal")) -> ()
                            }
                          }
                        }
                      }
                    }
                    n205 = Increment(x=w356) -> (x+1=w355:i32)
                  }
                  frame 1 {
                  }
                }
                n206 = feedback-in #2(w342) -> ()
                n207 = global read "Global_Variables.vi" "Auto Cal"() -> (w353:bool)
                n208 = case shown="True" w353 {
                  tunnel: w352 -> [w393 w396]
                  tunnel: [w392 w395] -> w349
                  tunnel: [w391 w394] -> w347
                  frame False {
                    n209 = call "Scan Hydra - Cal - Manual.vi"("error in"=w393) -> ("error out"=w392:errorcluster, "next scan"=w391:dbl[])  [unwired: 1 in]
                  }
                  frame True {
                    n210 = call "Scan Hydra - Cal - Auto.vi"("error in"=w396) -> ("error out"=w395:errorcluster, "next scan"=w394:dbl[])  [unwired: 1 in]
                  }
                }
                n211 = Array Size(array=w347) -> (size(s)=w351:i32)
                n212 = for {
                  N: w351 -> [_]
                  tunnel: w347 -> [w390]
                  tunnel: [w380] -> w350 mode=indexing
                  shift-right: [w389] -> w348
                  shift-left: w349 -> [w389]
                  i -> [w387]
                  n213 = global read "Global_Variables.vi" "Cal Channel"() -> (w388:dbl[])
                  n214 = Index Array(array=w388, index=w387) -> (element=w386:dbl)
                  n215 = Index Array(array=w390, index=w387) -> (element=w384:dbl)
                  n216 = To Long Integer(number=w386) -> (32bit integer=w385:i32)
                  n217 = Number To Decimal String(number=w385) -> (decimal integer string=w382:string)  [unwired: 1 in]
                  n218 = Number To Fractional String(number=w384, precision (6)=i16 4) -> (F-format string=w381:string)  [unwired: 2 in]
                  n219 = Build Array(w382, w381) -> (w380:string[])
                }
                "Data" <- w350
              }
              event "Cal Add": Value Change {
                n220 = event-data() -> ()  [unwired: 1 in, 1 out]
                n221 = case shown="True" "Cal Add" {
                  tunnel: w401 -> [w405 w410]
                  tunnel: [w405 w409] -> w400
                  tunnel: [enum16{"Minimum", "Maximum", "Calculations"}."Minimum" w406] -> w399
                  tunnel: [T1."Calibration" T1."Calibration"] -> w398
                  tunnel: w397 -> [_ w407]
                  frame False {
                  }
                  frame True {
                    n222 = global read "Global_Variables.vi" "Auto Cal"() -> (w411:bool)
                    n223 = case shown="True" w411 {
                      tunnel: w410 -> [w431 w459]
                      tunnel: [w413 w449] -> w409
                      frame False {
                        n224 = global read "Global_Variables.vi" "Cal Channel"() -> (w428:dbl[])
                        n225 = call "Scan Hydra - Cal - Manual.vi"("error in"=w431) -> ("error out"=w429:errorcluster, "next scan"=w427:dbl[])  [unwired: 1 in]
                        n226 = Array Size(array=w427) -> (size(s)=w430:i32)
                        n227 = for {
                          N: w430 -> [_]
                          shift-right: [w437] -> w425
                          shift-left: w429 -> [w437]
                          tunnel: w428 -> [w446]
                          tunnel: w427 -> [w445]
                          tunnel: [w439] -> w412 mode=indexing
                          tunnel: [w438] -> w426 mode=indexing
                          i -> [w444]
                          n228 = Index Array(array=w446, index=w444) -> (element=w443:dbl)
                          n229 = Index Array(array=w445, index=w444) -> (element=w439:dbl)
                          n230 = To Long Integer(number=w443) -> (32bit integer=w442:i32)
                          n231 = Number To Decimal String(number=w442) -> (decimal integer string=w441:string)  [unwired: 1 in]
                          n232 = Number To Fractional String(number=w439) -> (F-format string=w440:string)  [unwired: 3 in]
                          n233 = Build Array(w441, w440) -> (w438:string[])
                        }
                        n234 = global write "Global_Variables.vi" "Cal - Min Val"(w412) -> ()
                        n235 = local write "Data"(w426) -> ()
                        n236 = Open VI Reference(vi path=path "Min_Max_Entry.vi", error in (no error)=w425) -> (vi reference=w422:refnum<vi>, error out=w423:errorcluster)  [unwired: 4 in]
                        n237 = invoke class="VI" method="FP.Open"(reference=w422, error in=w423, "Activate"=TRUE ("Activate?")) -> (reference out=w419:refnum<vi>, error out=w420:errorcluster)  [unwired: 2 in, 3 out]
                        n238 = invoke class="VI" method="Run VI"(reference=w419, error in=w420, "Wait until done"=TRUE ("Wait Until Done")) -> (reference out=w416:refnum<vi>, error out=w417:errorcluster)  [unwired: 2 in, 3 out]
                        n239 = local read "Cal Add"() -> (w415:bool)
                        n240 = Close Reference(reference=w416, error in (no error)=w417) -> (error out=w414:errorcluster)
                        n241 = case shown="True" w415 {
                          tunnel: w414 -> [w432 w436]
                          tunnel: [w432 w436] -> w413
                          frame False {
                          }
                          frame True {
                            n242 = global read "Global_Variables.vi" "Min Max Ring"() -> (w434:u16)
                            n243 = local write "Cal Add"(FALSE ("Cal Add")) -> ()
                            n244 = Increment(x=w434) -> (x+1=w433:u16)
                            n245 = global write "Global_Variables.vi" "Min Max Ring"(w433) -> ()
                          }
                        }
                      }
                      frame True {
                        n246 = call "Scan Hydra - Cal - Auto.vi"("error in"=w459) -> ("error out"=w458:errorcluster, "next scan"=w453:dbl[])  [unwired: 1 in]
                        n247 = global read "Global_Variables.vi" "Cal Channel"() -> (w455:dbl[])
                        n248 = Array Size(array=w453) -> (size(s)=w457:i32)
                        n249 = Decrement(x=w457) -> (x-1=w456:i32)
                        n250 = for {
                          N: w456 -> [_]
                          shift-right: [w473] -> w450
                          shift-left: w458 -> [w473]
                          tunnel: w453 -> [w474]
                          tunnel: w455 -> [w471]
                          tunnel: [w467] -> w448 mode=indexing
                          tunnel: [w464] -> w454 mode=indexing
                          i -> [w472]
                          n251 = Increment(x=w472) -> (x+1=w463:i32)
                          n252 = Index Array(array=w474, index=w463) -> (element=w467:dbl)
                          n253 = Index Array(array=w471, index=w463) -> (element=w469:dbl)
                          n254 = To Long Integer(number=w469) -> (32bit integer=w470:i32)
                          n255 = Number To Decimal String(number=w470) -> (decimal integer string=w466:string)  [unwired: 1 in]
                          n256 = Number To Fractional String(number=w467, precision (6)=i16 4) -> (F-format string=w465:string)  [unwired: 2 in]
                          n257 = Build Array(w466, w465) -> (w464:string[])
                        }
                        n258 = local write "Data"(w454) -> ()
                        n259 = global write "Global_Variables.vi" "Cal - Min Val"(w448) -> ()
                        n260 = Index Array(array=w453, index=0) -> (element=w447:dbl)
                        n261 = global write "Global_Variables.vi" "Cal - Minimum"(w447) -> ()
                        n262 = local read "Cal Add"() -> (w451:bool)
                        n263 = case shown="True" w451 {
                          tunnel: w450 -> [w460 w461]
                          tunnel: [w460 w461] -> w449
                          frame False {
                          }
                          frame True {
                            n264 = local write "Cal Add"(FALSE ("Cal Add")) -> ()
                          }
                        }
                      }
                    }
                    n265 = Increment(x=w407) -> (x+1=w406:enum16{"Minimum", "Maximum", "Calculations"})
                  }
                }
              }
            }
          }
          frame "Maximum" {
            n266 = event shown="[1] \"Add Button\": Value Change" {
              selector: _ -> [_ _]
              dyn-events: _ -> [_ _]
              timeout: 1000 -> [_ _]
              tunnel: w479 -> [w481 w509]
              tunnel: w478 -> [w484 w510]
              tunnel: [w483 w508] -> w477
              tunnel: [T1."Calibration" w506] -> w476
              tunnel: [w481 w507] -> w475
              event Timeout {
                n267 = event-data() -> ()  [unwired: 1 in, 1 out]
                n268 = global read "Global_Variables.vi" "Auto Cal"() -> (w485:bool)
                n269 = case shown="True" w485 {
                  tunnel: w484 -> [w502 w505]
                  tunnel: [w501 w504] -> w487
                  tunnel: [w500 w503] -> w488
                  frame False {
                    n270 = call "Scan Hydra - Cal - Manual.vi"("error in"=w502) -> ("error out"=w501:errorcluster, "next scan"=w500:dbl[])  [unwired: 1 in]
                  }
                  frame True {
                    n271 = call "Scan Hydra - Cal - Auto.vi"("error in"=w505) -> ("error out"=w504:errorcluster, "next scan"=w503:dbl[])  [unwired: 1 in]
                  }
                }
                n272 = Array Size(array=w488) -> (size(s)=w486:i32)
                n273 = for {
                  N: w486 -> [_]
                  tunnel: w488 -> [w499]
                  tunnel: [w489] -> _ mode=indexing
                  shift-right: [w498] -> w483
                  shift-left: w487 -> [w498]
                  i -> [w496]
                  n274 = global read "Global_Variables.vi" "Cal Channel"() -> (w497:dbl[])
                  n275 = Index Array(array=w497, index=w496) -> (element=w495:dbl)
                  n276 = Index Array(array=w499, index=w496) -> (element=w493:dbl)
                  n277 = To Long Integer(number=w495) -> (32bit integer=w494:i32)
                  n278 = Number To Decimal String(number=w494) -> (decimal integer string=w491:string)  [unwired: 1 in]
                  n279 = Number To Fractional String(number=w493, precision (6)=i16 4) -> (F-format string=w490:string)  [unwired: 2 in]
                  n280 = Build Array(w491, w490) -> (w489:string[])
                }
              }
              event "Add Button": Value Change {
                n281 = event-data() -> ()  [unwired: 1 in, 1 out]
                n282 = local read "Cal Add"() -> (w511:bool)
                n283 = case shown="True" w511 {
                  tunnel: w510 -> [w514 w519]
                  tunnel: w509 -> [w513 w517]
                  tunnel: [w514 w515] -> w508
                  tunnel: [w513 w516] -> w507
                  tunnel: [T1."Calibration" w518] -> w506
                  frame False {
                  }
                  frame True {
                    n284 = global read "Global_Variables.vi" "Auto Cal"() -> (w520:bool)
                    n285 = case shown="True" w520 {
                      tunnel: w519 -> [w524 w560]
                      tunnel: [T1."Calibration" T1."Calibration"] -> w518
                      tunnel: [w521 w557] -> w515
                      frame False {
                        n286 = global read "Global_Variables.vi" "Cal Channel"() -> (w538:dbl[])
                        n287 = call "Scan Hydra - Cal - Manual.vi"("error in"=w524) -> ("error out"=w539:errorcluster, "next scan"=w537:dbl[])  [unwired: 1 in]
                        n288 = Array Size(array=w537) -> (size(s)=w540:i32)
                        n289 = for {
                          N: w540 -> [_]
                          shift-right: [w547] -> w535
                          shift-left: w539 -> [w547]
                          tunnel: w538 -> [w556]
                          tunnel: w537 -> [w555]
                          tunnel: [w549] -> w528 mode=indexing
                          tunnel: [w548] -> w536 mode=indexing
                          i -> [w554]
                          n290 = Index Array(array=w556, index=w554) -> (element=w553:dbl)
                          n291 = Index Array(array=w555, index=w554) -> (element=w549:dbl)
                          n292 = To Long Integer(number=w553) -> (32bit integer=w552:i32)
                          n293 = Number To Decimal String(number=w552) -> (decimal integer string=w551:string)  [unwired: 1 in]
                          n294 = Number To Fractional String(number=w549) -> (F-format string=w550:string)  [unwired: 3 in]
                          n295 = Build Array(w551, w550) -> (w548:string[])
                        }
                        n296 = global write "Global_Variables.vi" "Cal - Max Val"(w528) -> ()
                        n297 = local write "Data"(w536) -> ()
                        n298 = Open VI Reference(vi path=path "Min_Max_Entry.vi", error in (no error)=w535) -> (vi reference=w533:refnum<vi>, error out=w534:errorcluster)  [unwired: 4 in]
                        n299 = invoke class="VI" method="FP.Open"(reference=w533, error in=w534, "Activate"=TRUE ("Activate?")) -> (reference out=w531:refnum<vi>, error out=w532:errorcluster)  [unwired: 2 in, 3 out]
                        n300 = invoke class="VI" method="Run VI"(reference=w531, error in=w532, "Wait until done"=TRUE ("Wait Until Done")) -> (reference out=w529:refnum<vi>, error out=w530:errorcluster)  [unwired: 2 in, 3 out]
                        n301 = local read "Cal Add"() -> (w523:bool)
                        n302 = Close Reference(reference=w529, error in (no error)=w530) -> (error out=w522:errorcluster)
                        n303 = case shown="True" w523 {
                          tunnel: w522 -> [w542 w545]
                          tunnel: [w542 w545] -> w521
                          frame False {
                          }
                          frame True {
                            n304 = global read "Global_Variables.vi" "Min Max Ring"() -> (w544:u16)
                            n305 = local write "Cal Add"(FALSE ("Cal Add")) -> ()
                            n306 = Decrement(x=w544) -> (x-1=w543:u16)
                            n307 = global write "Global_Variables.vi" "Min Max Ring"(w543) -> ()
                          }
                        }
                      }
                      frame True {
                        n308 = call "Scan Hydra - Cal - Auto.vi"("error in"=w560) -> ("error out"=w569:errorcluster, "next scan"=w564:dbl[])  [unwired: 1 in]
                        n309 = global read "Global_Variables.vi" "Cal Channel"() -> (w566:dbl[])
                        n310 = Array Size(array=w564) -> (size(s)=w568:i32)
                        n311 = Decrement(x=w568) -> (x-1=w567:i32)
                        n312 = for {
                          N: w567 -> [_]
                          shift-right: [w584] -> w558
                          shift-left: w569 -> [w584]
                          tunnel: w564 -> [w585]
                          tunnel: w566 -> [w582]
                          tunnel: [w578] -> w563 mode=indexing
                          tunnel: [w575] -> w565 mode=indexing
                          i -> [w583]
                          n313 = Increment(x=w583) -> (x+1=w574:i32)
                          n314 = Index Array(array=w585, index=w574) -> (element=w578:dbl)
                          n315 = Index Array(array=w582, index=w574) -> (element=w580:dbl)
                          n316 = To Long Integer(number=w580) -> (32bit integer=w581:i32)
                          n317 = Number To Decimal String(number=w581) -> (decimal integer string=w577:string)  [unwired: 1 in]
                          n318 = Number To Fractional String(number=w578, precision (6)=i16 4) -> (F-format string=w576:string)  [unwired: 2 in]
                          n319 = Build Array(w577, w576) -> (w575:string[])
                        }
                        n320 = local write "Data"(w565) -> ()
                        n321 = global write "Global_Variables.vi" "Cal - Max Val"(w563) -> ()
                        n322 = Index Array(array=w564, index=0) -> (element=w562:dbl)
                        n323 = global write "Global_Variables.vi" "Cal - Maximum"(w562) -> ()
                        n324 = local read "Cal Add"() -> (w559:bool)
                        n325 = case shown="True" w559 {
                          tunnel: w558 -> [w571 w573]
                          tunnel: [w571 w573] -> w557
                          frame False {
                          }
                          frame True {
                            n326 = local write "Cal Add"(FALSE ("Cal Add")) -> ()
                          }
                        }
                      }
                    }
                    n327 = Increment(x=w517) -> (x+1=w516:enum16{"Minimum", "Maximum", "Calculations"})
                  }
                }
              }
            }
          }
          frame "Calculations" {
            n328 = call "Cal_Calculations.vi"("Error In"=w588) -> ("Error Out"=w587:errorcluster)
            n329 = global write "Global_Variables.vi" "Cal complete"(TRUE ("Cal complete")) -> ()
            n330 = Wait (ms)(milliseconds to wait=u32 2500) -> ()  [unwired: 1 out]
          }
        }
        n331 = feedback-in #1(w332) -> ()
        n332 = local write "Status"("Calibration" ("Status")) -> ()
      }
      frame "Test" {
        n333 = global read "Global_Variables.vi" "Cal complete"() -> (w595:bool)
        n334 = case shown="True" w595 {
          tunnel: w594 -> [w598 w610]
          tunnel: [w598 w602] -> w593
          tunnel: [T1."Wait for Config" w600] -> w592
          frame False {
          }
          frame True {
            n335 = global read "Global_Variables.vi" "Channel Num"() -> (w606:dbl[])
            n336 = call "Scan Hydra - Test.vi"("error in"=w610) -> ("error out"=w608:errorcluster, "next scan"=w607:dbl[])  [unwired: 1 in]
            n337 = Array Size(array=w606) -> (size(s)=w609:i32)
            n338 = for {
              N: w609 -> [_]
              tunnel: w607 -> [w623]
              tunnel: w606 -> [w624]
              shift-right: [w621] -> w604
              shift-left: w608 -> [w621]
              tunnel: [w615] -> w605 mode=indexing
              tunnel: [w614] -> w603 mode=indexing
              i -> [w622]
              n339 = Index Array(array=w624, index=w622) -> (element=w620:dbl)
              n340 = Index Array(array=w623, index=w622) -> (element=w618:dbl)
              n341 = To Long Integer(number=w620) -> (32bit integer=w619:i32)
              n342 = Number To Decimal String(number=w619) -> (decimal integer string=w616:string)  [unwired: 1 in]
              n343 = Number To Fractional String(number=w618, precision (6)=i16 4) -> (F-format string=w614:string)  [unwired: 2 in]
              n344 = Build Array(w616, w614) -> (w615:string[])
            }
            n345 = local write "Data"(w605) -> ()
            n346 = call "Report_Data.vi"("Error In"=w604, "Values"=w603) -> ("Error Out"=w602:errorcluster)  [unwired: 1 in]
            n347 = local write "Status"("Performing Test" ("Status")) -> ()
            n348 = case shown="True" "Stop Test" {
              tunnel: [T1."Test" T1."Initialize"] -> w600
              frame False {
              }
              frame True {
                n349 = local write "Stop Test"(FALSE ("Stop Test")) -> ()
              }
            }
          }
        }
      }
      frame "Close" {
        n350 = local write "Status"("Closing LabView" ("Status")) -> ()
        n351 = Wait (ms)(milliseconds to wait=u32 2500) -> ()  [unwired: 1 out]
      }
    }
    n352 = call <vilib>:"General Error Handler.vi"("error in (no error)"=w16) -> ("code out"=→"Error Code":i32, "source out"=w12:string, "message"=w8:string, "error out"=w15:errorcluster)  [unwired: 10 in, 1 out]
    n353 = Build Array("Error Source:", w12, w10, "-------------------------------", w10, "Error Description:", w8) -> (w7:string[])
    n354 = Array To Spreadsheet String(delimiter (Tab)="\r\n", array=w7, 3:"" ("format string")) -> (spreadsheet string=→"Error Description":string)
  }
